vi "Perform convolution.vi"(8 "Sample stream":cdb[](array[numeric]) format="%.2f", 10 "Pulse Shaping Filter Coefficients":cdb[](array[numeric]) format="%.2f") -> (2 "Filtered sample stream":cdb[](array[numeric]))   [LabVIEW 2011]
uses:
  <vilib>/Analysis/2dsp.llb/1D Convolution (CDB).vi
  <vilib>/Analysis/NI_AALPro.lvlib
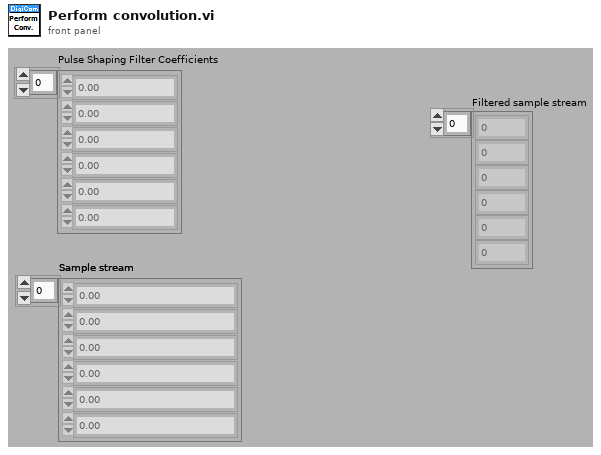
[diagram p1: front panel]
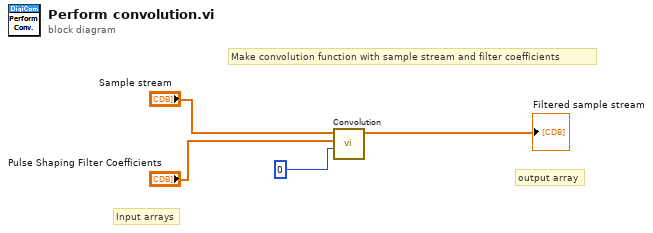
[diagram p0: block diagram]
diagram:
  # "output array"
  # "Input arrays"
  # "Make convolution function with sample stream and filter coefficients"
  n1 = call-poly <vilib>:"Convolution.vi"("algorithm"=0, "Y"="Pulse Shaping Filter Coefficients", "X"="Sample stream") -> ("X * Y"=→"Filtered sample stream":cdb[])  [unwired: 7 in, 1 out]
